vi "Configure Bursted Generation.vi"(0 "RFSG handle":refnum<k15>, 5 "Waveform":T1={"Name"="Wfm", "Data"=refnum, "Signal Bandwidth (Hz)"=0.0, "PAPR (dB)"=0.0, "Burst Length (s)"=0.0, "Sample Rate"=0.0, "Burst Start Locations"=[], "Burst Stop Locations"=[], "Idle Duration Present?"=FALSE, "Runtime Scaling"=0.0, "Script"=""} {"Runtime Scaling" format="%#_6p"; "Sample Rate" format="%#_6p"; "Burst Length (s)" format="%#_6p"; "PAPR (dB)" format="%.2f"; "Signal Bandwidth (Hz)" format="%#_6p"}, 7 "Waveform Timing Configuration":T4={"Duty Cycle (%)"=50.0, "Pre-Burst Time (s)"=1e-06, "Post-Burst Time (s)"=1e-06, "Burst Start Trigger Export"="PXI_Trig0"} {"Post-Burst Time (s)" format="%#_6p"; "Pre-Burst Time (s)" format="%#_6p"; "Duty Cycle (%)" min=1.0 max=100.0 step=1.0 format="%#_2d%%"}, 9 "PAEN Configuration":T2={"PAEN Mode"=enum."Dynamic", "PA Enable Trigger Export Terminal"="PFI0", "PA Enable Trigger Mode"=23001, "Command Enable Time (s)"=0.0, "Command Disable Time (s)"=0.0} {"PA Enable Trigger Mode" items=["Pulse"=23000, "Toggle"=23001]; "Command Disable Time (s)" format="%#_6p"; "Command Enable Time (s)" format="%#_6p"}, 11 "error in":errorcluster) -> (4 "RFSG handle out":refnum<k15>, 6 "Waveform out":T1={"Name"="Wfm", "Data"=refnum, "Signal Bandwidth (Hz)"=0.0, "PAPR (dB)"=0.0, "Burst Length (s)"=0.0, "Sample Rate"=0.0, "Burst Start Locations"=[], "Burst Stop Locations"=[], "Idle Duration Present?"=FALSE, "Runtime Scaling"=0.0, "Script"=""} {"Runtime Scaling" format="%#_6p"; "Sample Rate" format="%#_6p"; "Burst Length (s)" format="%#_6p"; "PAPR (dB)" format="%.2f"; "Signal Bandwidth (Hz)" format="%#_6p"}, 8 "Generation Period (s)":dbl format="%#_6p", 15 "error out":errorcluster)   [LabVIEW 2019, in "SG.lvlib"]
doc: "Configures the generator to generate the waveform plus idle time continuously for Dynamic EVM test cases. Also configures triggering or pulsing settings to control the DUT. Use <b>Abort Generation</b> to abort generation to always ensure that the DUT state is returned to the initial state."
uses:
  SG.lvlib
  Common/Waveform.ctl
  Typedefs/Waveform Timing Configuration.ctl
  <instrlib>/niRFSG/niRFSG.llb/niRFSG Exported Signal Destinations.ctl
  Typedefs/PAEN Configuration.ctl
  <instrlib>/niRFSG/niRFSG.llb/niRFSG Signal Names.ctl
  <instrlib>/niRFSG/niRFSG.llb/niRFSG Signal Identifiers.ctl
  <instrlib>/niRFSG/niRFSG.llb/niRFSG Script Trigger IDs.ctl
  <vilib>/Utility/error.llb/Error Cluster From Error Code.vi
  <instrlib>/niRFSG/niRFSG.llb/niRFSG Configure Script Trigger Software.vi
  <vilib>/ErrorRing/Error Ring.xnode
  Common/Common.lvlib
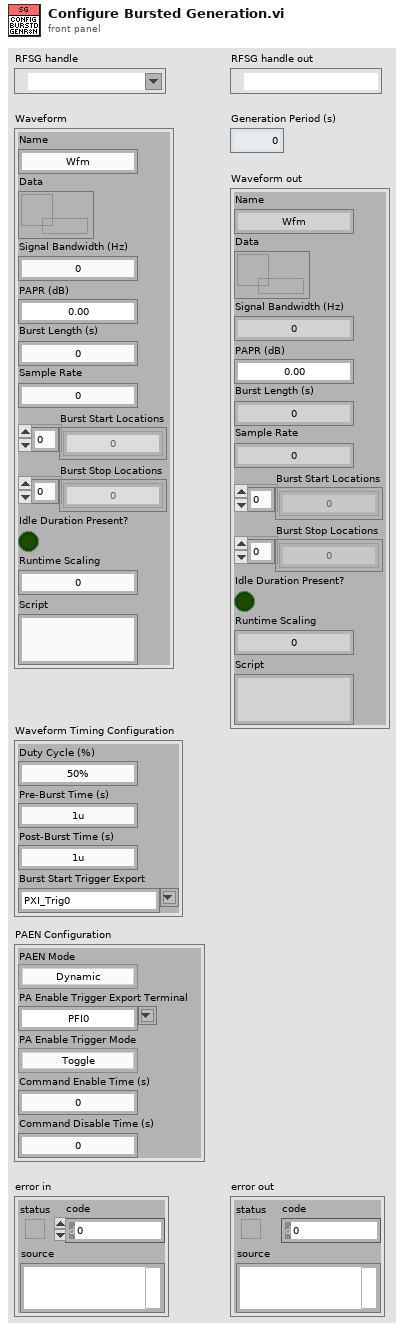
[diagram p1: front panel]
types:
  T1 = typedef "Common.lvlib/Waveform.ctl" = cluster{"Name":string, "Data":refnum<data-value>, "Signal Bandwidth (Hz)":dbl, "PAPR (dB)":dbl, "Burst Length (s)":dbl, "Sample Rate":dbl, "Burst Start Locations":i32[], "Burst Stop Locations":i32[], "Idle Duration Present?":bool, "Runtime Scaling":dbl, "Script":string}
  T2 = typedef "SG.lvlib/PAEN Configuration.ctl" = cluster{"PAEN Mode":enum16{"Disabled", "Static", "Dynamic"}, "PA Enable Trigger Export Terminal":T3, "PA Enable Trigger Mode":i32, "Command Enable Time (s)":dbl, "Command Disable Time (s)":dbl}
  T3 = typedef "niRFSG Exported Signal Destinations.ctl" = string
  T4 = typedef "SG.lvlib/Waveform Timing Configuration.ctl" = cluster{"Duty Cycle (%)":dbl, "Pre-Burst Time (s)":dbl, "Post-Burst Time (s)":dbl, "Burst Start Trigger Export":T3}
  T5 = typedef "niRFSG Script Trigger IDs.ctl" = string
  T6 = typedef "niRFSG Signal Identifiers.ctl" = string
  T7 = typedef "niRFSG Signal Names.ctl" = i32
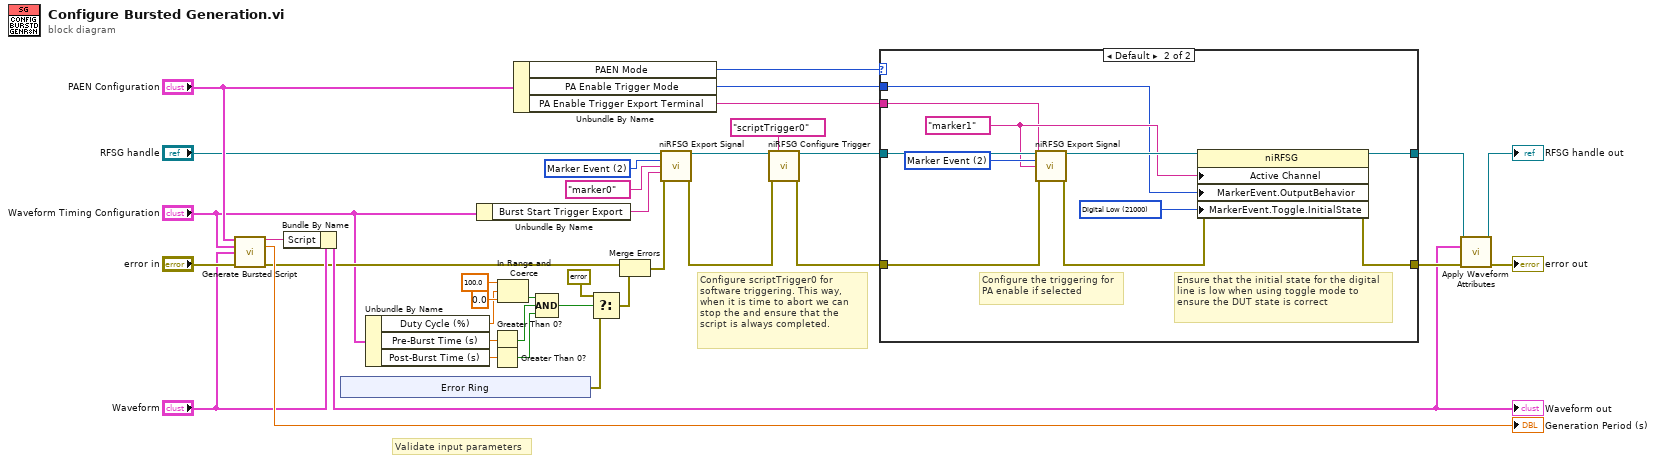
[diagram p0: block diagram]
diagram:
  w26 = T7 2 items=["Start Trigger", "Script Trigger", "Marker Event", "Ref Clock", "Started Event", "Done Event", "Configuration List Step Trigger", "Configuration Settled Event"] ("signal")
  # "Validate input parameters"
  # "Configure scriptTrigger0 for software triggering. This way, when it is time to abort we can stop the and ensure that the script is always completed."
  n1 = call "Generate Bursted Script.vi"("PAEN Config"="PAEN Configuration", "Waveform Timing Configuration"="Waveform Timing Configuration", "Waveform"="Waveform", "error in (no error)"="error in") -> ("Script"=w20:string, "Generation Period (s)"=→"Generation Period (s)":dbl, "error out"=w3:errorcluster)  [unwired: 9 in]
  n2 = Bundle By Name(cluster="Waveform", "Script"=w20) -> (w16:T1)
  "Waveform out" <- w16
  n3 = xnode "Error Ring"() -> ("error out"=w6:errorcluster)
  n4 = Unbundle By Name("Waveform Timing Configuration") -> ("Duty Cycle (%)"=w13:dbl, "Pre-Burst Time (s)"=w12:dbl, "Post-Burst Time (s)"=w11:dbl)
  n5 = Unbundle By Name("Waveform Timing Configuration") -> ("Burst Start Trigger Export"=w24:T3)
  n6 = Greater Than 0?(x=w12) -> (x > 0?=w9:bool)
  n7 = Greater Than 0?(x=w11) -> (x > 0?=w8:bool)
  n8 = In Range and Coerce(upper limit=100.0, x=w13, lower limit=0.0) -> (In Range?=w10:bool)  [unwired: 1 out]
  n9 = Unbundle By Name("PAEN Configuration") -> ("PAEN Mode"=w29:enum16{"Disabled", "Static", "Dynamic"}, "PA Enable Trigger Mode"=w28:i32, "PA Enable Trigger Export Terminal"=w27:T3)
  n10 = Compound Arithmetic op=AND(w10, w9, w8) -> (w7:bool)
  n11 = Select(t=errorcluster {"status"=FALSE, "code"=0, "source"=""} ("error constant"), s=w7, f=w6) -> (s? t:f=w5:errorcluster)
  n12 = Merge Errors(w3, w5) -> (w4:errorcluster)
  n13 = call <instrlib>:"niRFSG Export Signal.vi"("instrument handle"="RFSG handle", "signal"=w26, "signal identifier"=T6 "marker0", "output terminal"=w24, "error in"=w4) -> ("instrument handle out"=w22:refnum<k15>, "error out"=w36:errorcluster)  [unwired: 9 in]
  n14 = call-poly <instrlib>:"niRFSG Configure Trigger.vi"("instrument handle"=w22, "trigger id"=T5 "scriptTrigger0", "error in"=w36) -> ("instrument handle out"=w21:refnum<k15>, "error out"=w35:errorcluster)  [unwired: 11 in]
  n15 = case "Configure the triggering for PA enable if selected" shown="Default" w29 {
    tunnel: [w39 w48] -> w34
    tunnel: w35 -> [w39 w50]
    tunnel: [w38 w41] -> w17
    tunnel: w21 -> [w38 w47]
    tunnel: w28 -> [_ w43]
    tunnel: w27 -> [_ w42]
    frame "Disabled" {
    }
    frame Default {
      w40 = 21000 items=["Digital Low"=21000, "Digital High"=21001] ("Events:Marker:Toggle:Initial State")
      w44 = T6 "marker1" ("signal identifier")
      w45 = T7 2 items=["Start Trigger", "Script Trigger", "Marker Event", "Ref Clock", "Started Event", "Done Event", "Configuration List Step Trigger", "Configuration Settled Event"] ("signal")
      # "Ensure that the initial state for the digital line is low when using toggle mode to ensure the DUT state is correct"
      # "Configure the triggering for PA enable if selected"
      n16 = call <instrlib>:"niRFSG Export Signal.vi"("instrument handle"=w47, "signal"=w45, "signal identifier"=w44, "output terminal"=w42, "error in"=w50) -> ("instrument handle out"=w46:refnum<k15>, "error out"=w49:errorcluster)  [unwired: 9 in]
      n17 = property class="niRFSG"(reference=w46, error in=w49, "Active Channel"=w44, "MarkerEvent.OutputBehavior"=w43, "MarkerEvent.Toggle.InitialState"=w40) -> (reference out=w41:refnum<k15>, error out=w48:errorcluster)
    }
  }
  n18 = call "Apply Waveform Attributes.vi"("RFSG Session In"=w17, "Waveform"=w16, "error in (no error)"=w34) -> ("RFSG Session Out"=→"RFSG handle out":refnum<k15>, "error out"=→"error out":errorcluster)  [unwired: 11 in]
